vi "Init Debug.vi"(8 "error in (no error)":errorcluster, 11 "Volatus Core in":refnum<class "Volatus Core.lvclass">) -> (0 "error out":errorcluster, 3 "Volatus Core out":refnum<class "Volatus Core.lvclass">)   [LabVIEW 2020, in "Volatus.lvlib" / "Volatus Core.lvclass"]
uses:
  Volatus Core.lvclass
  Volatus Core.lvclass/Volatus Core.ctl
  Module/Module.lvclass
  C:/dev/lv20CE/relink/lv-volatus/Volatus/Module/Module.lvclass
  C:/dev/lv20CE/relink/lv-volatus/Volatus/Volatus Core/Volatus Core.lvclass
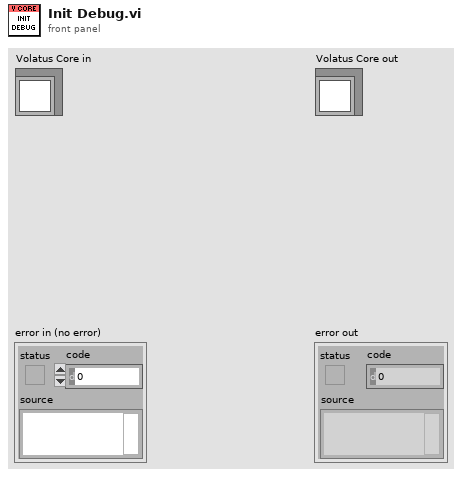
[diagram p1: front panel]
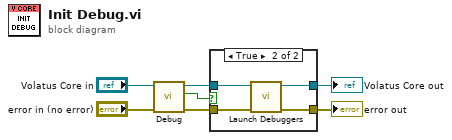
[diagram p0: block diagram]
diagram:
  n1 = call "Debug.vi"("Module in"="Volatus Core in") -> ("Debug"=w6:bool, "Module out"=w4:refnum<class "Volatus Core.lvclass">)  [unwired: 9 in]
  n2 = case shown="True" w6 {
    tunnel: w4 -> [w8 w12]
    tunnel: "error in (no error)" -> [w7 w10]
    tunnel: [w8 w11] -> w2
    tunnel: [w7 w9] -> w1
    frame False {
    }
    frame True {
      n3 = call "Launch Debuggers.vi"("error in (no error)"=w10, "Volatus Core in"=w12) -> ("error out"=w9:errorcluster, "Volatus Core out"=w11:refnum<class "Volatus Core.lvclass">)  [unwired: 8 in]
    }
  }
  "error out" <- w1
  "Volatus Core out" <- w2
